vi "Write Report to Excel.vi"(8 "error in (no error)":errorcluster, 10 "Row Data":T1, 11 "Excel Logger in":refnum<class "Excel Logger.lvclass">) -> (0 "error out":errorcluster, 3 "Excel Logger out":refnum<class "Excel Logger.lvclass">)   [LabVIEW 2016, in "generate report.lvlib"]
uses:
  generate report.lvlib
  core/Classes/Excel Logger/Excel Logger.lvclass
  core/Classes/Data Analyser Report/Data Analyser Report.lvclass
  C:/Users/w.figtree/Desktop/Work/4. Projects/3. In Progress Engineering Projects/EMA/src/core/Classes/Excel Interface/Excel Sheet/Excel Sheet.lvclass
  core/Classes/Excel Interface/Excel Sheet/Write to Cell - Variant.vi
  core/Classes/Excel Interface/Excel Sheet/Excel Sheet.lvclass
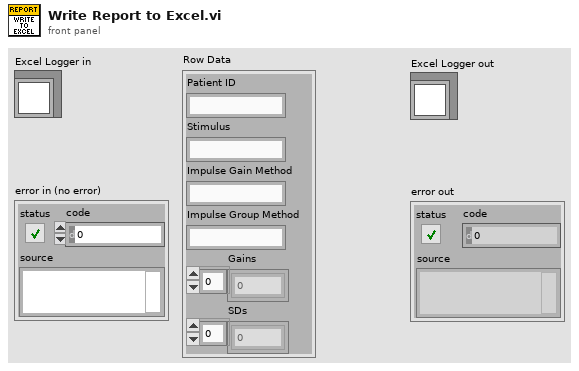
[diagram p1: front panel]
types:
  T1 = cluster{"Patient ID":string, "Stimulus":string, "Impulse Gain Method":string, "Impulse Group Method":string, "Gains":dbl[], "SDs":dbl[]}
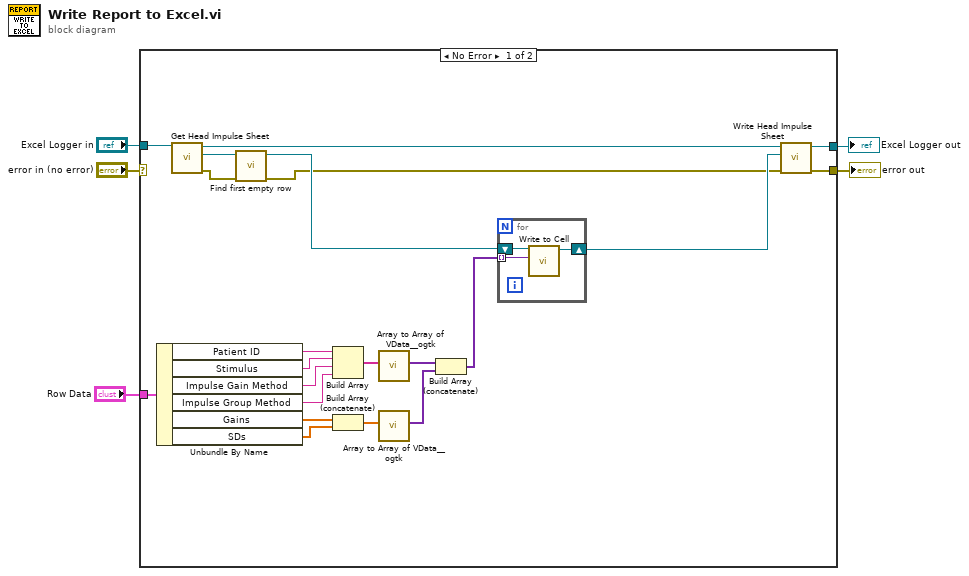
[diagram p0: block diagram]
diagram:
  n1 = case shown="No Error" "error in (no error)" {
    selector: "error in (no error)" -> [_ w30]
    tunnel: "Excel Logger in" -> [w26 w31]
    tunnel: "Row Data" -> [w23 _]
    tunnel: [w7 w30] -> w1
    tunnel: [w6 w31] -> w2
    frame No Error {
      n2 = Unbundle By Name(w23) -> ("Patient ID"=w21:string, "Stimulus"=w20:string, "Impulse Gain Method"=w19:string, "Impulse Group Method"=w18:string, "Gains"=w17:dbl[], "SDs"=w16:dbl[])
      n3 = call "Get Head Impulse Sheet.vi"("Excel Logger in"=w26) -> ("error out"=w9:errorcluster, "Head Impulse"=w25:refnum<class "Data Analyser Report.lvclass">, "Excel Logger out"=w24:refnum<class "Excel Logger.lvclass">)  [unwired: 8 in]
      n4 = call-dynamic "Find first empty row.vi"("error in (no error)"=w9, "Excel Sheet in"=w25) -> ("error out"=w8:errorcluster, "Excel Sheet out"=w22:refnum<class "Data Analyser Report.lvclass">)  [unwired: 7 in, 1 out]
      n5 = Build Array(w21, w20, w19, w18) -> (w15:string[])
      n6 = Build Array (concatenate)(w17, w16) -> (w14:dbl[])
      n7 = call <userlib>:"Array to Array of VData__ogtk.vi"("MultiD Array"=w15) -> ("1D Array of Variants"=w13:variant[])  [unwired: 9 in, 1 out]
      n8 = call <userlib>:"Array to Array of VData__ogtk.vi"("MultiD Array"=w14) -> ("1D Array of Variants"=w12:variant[])  [unwired: 9 in, 1 out]
      n9 = Build Array (concatenate)(w13, w12) -> (w11:variant[])
      n10 = for {
        tunnel: w11 -> [w28] mode=indexing
        shift-right: [w27] -> w10
        shift-left: w22 -> [w29]
        n11 = call-poly "Write to Cell.vi"("Value"=w28, "Excel Sheet in"=w29) -> ("Excel Sheet out"=w27:refnum<class "Data Analyser Report.lvclass">)  [unwired: 9 in]
      }
      n12 = call "Write Head Impulse Sheet.vi"("error in (no error)"=w8, "Head Impulse"=w10, "Excel Logger in"=w24) -> ("error out"=w7:errorcluster, "Excel Logger out"=w6:refnum<class "Excel Logger.lvclass">)  [unwired: 7 in]
    }
    frame Error {
    }
  }
  "error out" <- w1
  "Excel Logger out" <- w2
